vi "CurrentConfig.vi"(0 "Current":bool, 1 "IP":string caption="IP地址") -> ()   [LabVIEW 2012]
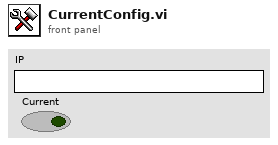
[diagram p1: front panel]
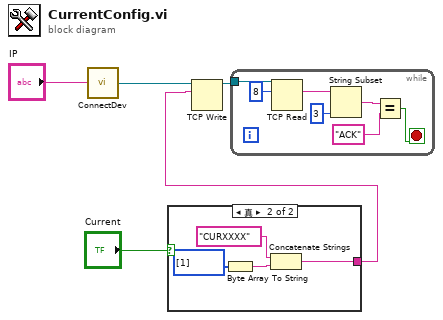
[diagram p0: block diagram]
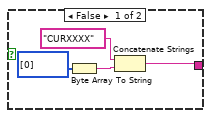
[diagram p2: hidden frame]
diagram:
  n1 = call "ConnectDev.vi"("IP."="IP") -> ("connection ID"=w1:refnum<k5>)
  n2 = case shown="真" "Current" {
    tunnel: [w6 w10] -> w4
    frame False {
      n3 = Byte Array To String(unsigned byte array=u8[] [0] ("无符号字节数组")) -> (string=w8:string)
      n4 = Concatenate Strings("CURXXXX" ("数据输入"), w8) -> (w6:string)
    }
    frame True {
      n5 = Byte Array To String(unsigned byte array=u8[] [1] ("无符号字节数组")) -> (string=w12:string)
      n6 = Concatenate Strings("CURXXXX" ("数据输入"), w12) -> (w10:string)
    }
  }
  n7 = TCP Write(connection ID=w1, data in=w4) -> (connection ID out=w5:refnum<k5>)  [unwired: 2 in, 2 out]
  n8 = while {
    tunnel: w5 -> [w20]
    stop <- w15 stop-if-true
    n9 = TCP Read(connection ID=w20, bytes to read=8 ("读取的字节")) -> (data out=w18:string)  [unwired: 3 in, 2 out]
    n10 = String Subset(string=w18, length (rest)=3 ("偏移量(0)")) -> (substring=w17:string)  [unwired: 1 in]
    n11 = Equal?(x=w17, y="ACK") -> (x = y?=w15:bool)
  }
